vi "HTML Hierarhy Ref.vi"(11 "Byte Stream File in":refnum<file>) -> (3 "Byte Stream File out":refnum<file>)   [LabVIEW 2014, in "lvprj2html.lvlib"]
uses:
  lvprj2html.lvlib
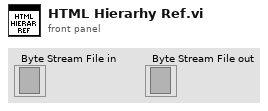
[diagram p1: front panel]
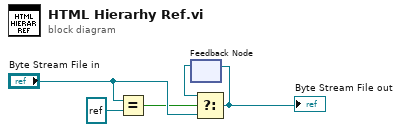
[diagram p0: block diagram]
diagram:
  n1 = Equal?(x="Byte Stream File in", y=refnum<file> refnum ("refnum out")) -> (x = y?=w2:bool)
  n2 = feedback #1() -> (w4:refnum<file>)  [unwired: 1 in]
  n3 = Select(t=w4, s=w2, f="Byte Stream File in") -> (s? t:f=w3:refnum<file>)
  "Byte Stream File out" <- w3
  n4 = feedback-in #1(w3) -> ()
